vi "删除预设波形.vi"(10 "波形点":cluster{"时间点":dbl, "幅值":dbl}, 11 "原预设波形":dbl[][](array[numeric])) -> (2 "删除后波形":dbl[][](array[numeric]))   [LabVIEW 2018]
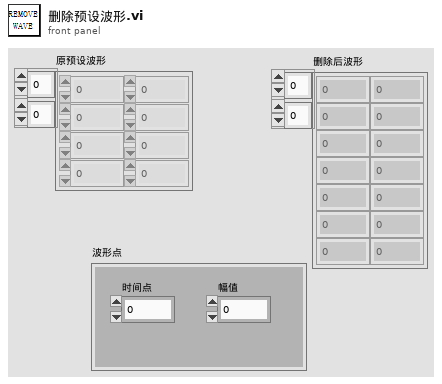
[diagram p1: front panel]
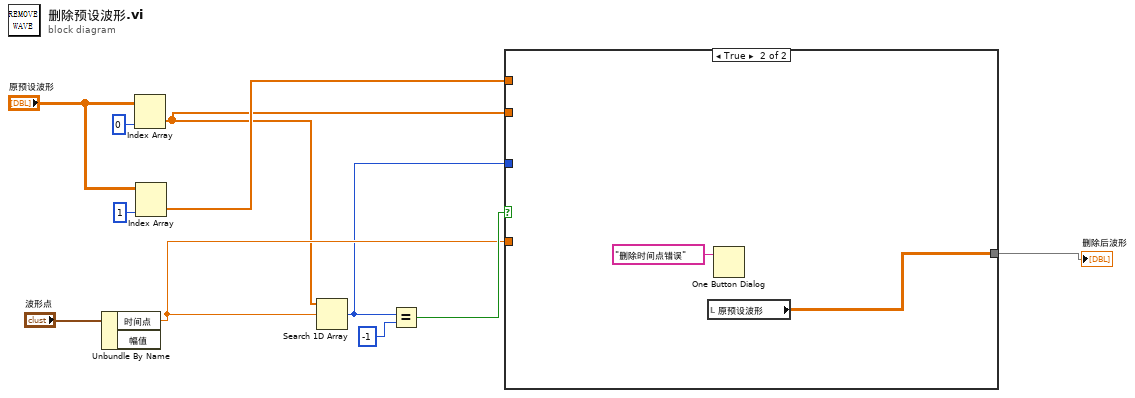
[diagram p0: block diagram]
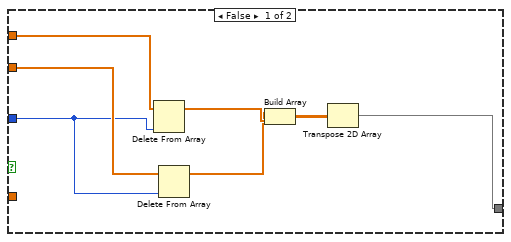
[diagram p2: hidden frame]
diagram:
  n1 = Unbundle By Name("波形点") -> ("时间点"=w7:dbl)  [unwired: 1 out]
  n2 = Index Array(array="原预设波形", index (col)=0 ("disabled index (col)")) -> (element=w2:dbl[])  [unwired: 1 in]
  n3 = Index Array(array="原预设波形", index (col)=1 ("disabled index (col)")) -> (element=w4:dbl[])  [unwired: 1 in]
  n4 = Search 1D Array(1D array=w2, element=w7) -> (index of element=w3:i32)  [unwired: 1 in]
  n5 = Equal?(x=w3, y=-1) -> (x = y?=w8:bool)
  n6 = case shown="True" w8 {
    tunnel: w7 -> [_ _]
    tunnel: [w15 w20] -> w6
    tunnel: w4 -> [w18 _]
    tunnel: w3 -> [w13 _]
    tunnel: w2 -> [w14 _]
    frame False {
      n7 = Delete From Array(array=w18, index=w13) -> (array with subset deleted=w17:dbl[])  [unwired: 1 in, 1 out]
      n8 = Delete From Array(array=w14, index=w13) -> (array with subset deleted=w12:dbl[])  [unwired: 1 in, 1 out]
      n9 = Build Array(w12, w17) -> (w16:dbl[][])
      n10 = Transpose 2D Array(2D array=w16) -> (transposed array=w15:dbl[][])
    }
    frame True {
      n11 = local read "原预设波形"() -> (w20:dbl[][])
      n12 = One Button Dialog(message="删除时间点错误") -> ()  [unwired: 1 in, 1 out]
    }
  }
  "删除后波形" <- w6
